vi "Get data.vi"(8 "error in (no error)":errorcluster, 10 "Seleccion":T1, 11 "url":string) -> (0 "error out":errorcluster, 2 "Variant":variant)   [LabVIEW 2018]
uses:
  Seleccion.ctl
  Valores venta almacen.ctl
  Valores Zapato.ctl
  Modelo color.ctl
  <vilib>/httpClient/LabVIEWHTTPClient.lvlib
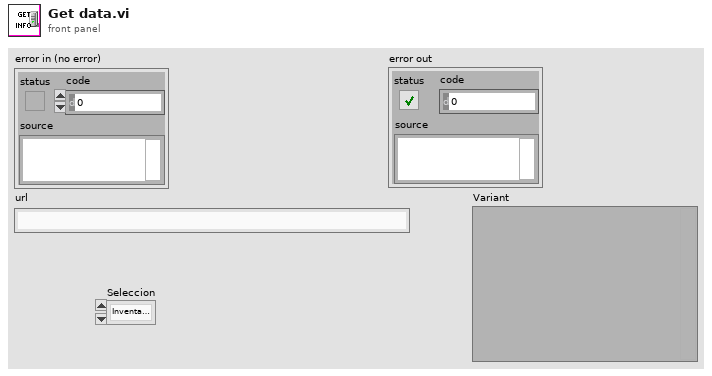
[diagram p1: front panel]
types:
  T1 = typedef "Seleccion.ctl" = enum16{"Inventario/ventas", "Zapatos", "Modelo/color"}
  T2 = typedef "Valores venta almacen.ctl" = cluster{"Cantidad":dbl, "Codigo":string, "Color":string, "Locacion/fecha":string, "Modelo":string, "Talla":string}
  T3 = typedef "Valores Zapato.ctl" = cluster{"Codigo":string, "Color":string, "Modelo":string, "Talla":string}
  T4 = typedef "Modelo color.ctl" = cluster{"Modelo/color":string}
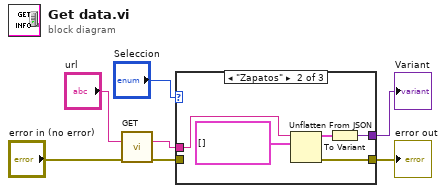
[diagram p0: block diagram]
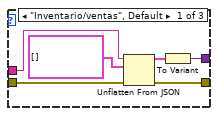
[diagram p2: hidden frame]
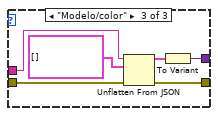
[diagram p3: hidden frame]
diagram:
  n1 = call <vilib>:"GET.vi"("url"="url", "error in (no error)"="error in (no error)") -> ("headers"=w1:string, "error out"=w5:errorcluster)  [unwired: 10 in, 2 out]
  n2 = case shown="\"Zapatos\"" "Seleccion" {
    tunnel: [w10 w17 w21] -> w4
    tunnel: [w9 w16 w20] -> w2
    tunnel: w5 -> [w11 _ w22]
    tunnel: w1 -> [w12 w14 w23]
    frame "Inventario/ventas", Default {
      n3 = Unflatten From JSON(JSON string=w12, type and defaults=T2[] [], error in (no error)=w11) -> (value=w13:T2[], error out=w10:errorcluster)  [unwired: 4 in]
      n4 = To Variant(anything=w13) -> (Variant=w9:variant)
    }
    frame "Zapatos" {
      n5 = Unflatten From JSON(JSON string=w14, type and defaults=T3[] []) -> (value=w18:T3[], error out=w17:errorcluster)  [unwired: 5 in]
      n6 = To Variant(anything=w18) -> (Variant=w16:variant)
    }
    frame "Modelo/color" {
      n7 = Unflatten From JSON(JSON string=w23, type and defaults=T4[] [], error in (no error)=w22) -> (value=w24:T4[], error out=w21:errorcluster)  [unwired: 4 in]
      n8 = To Variant(anything=w24) -> (Variant=w20:variant)
    }
  }
  "error out" <- w4
  "Variant" <- w2
